vi "BITMAPINFOHEADER.vi"(11 "Dimensions de l'image":i32[](array[numeric])) -> (3 "EN-TÊTE_FICHIER_BITMAP":u8[](array[numeric]))   [LabVIEW 2009]
panel:
  out "taille(s)":i32
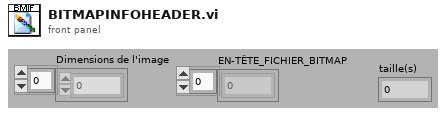
[diagram p1: front panel]
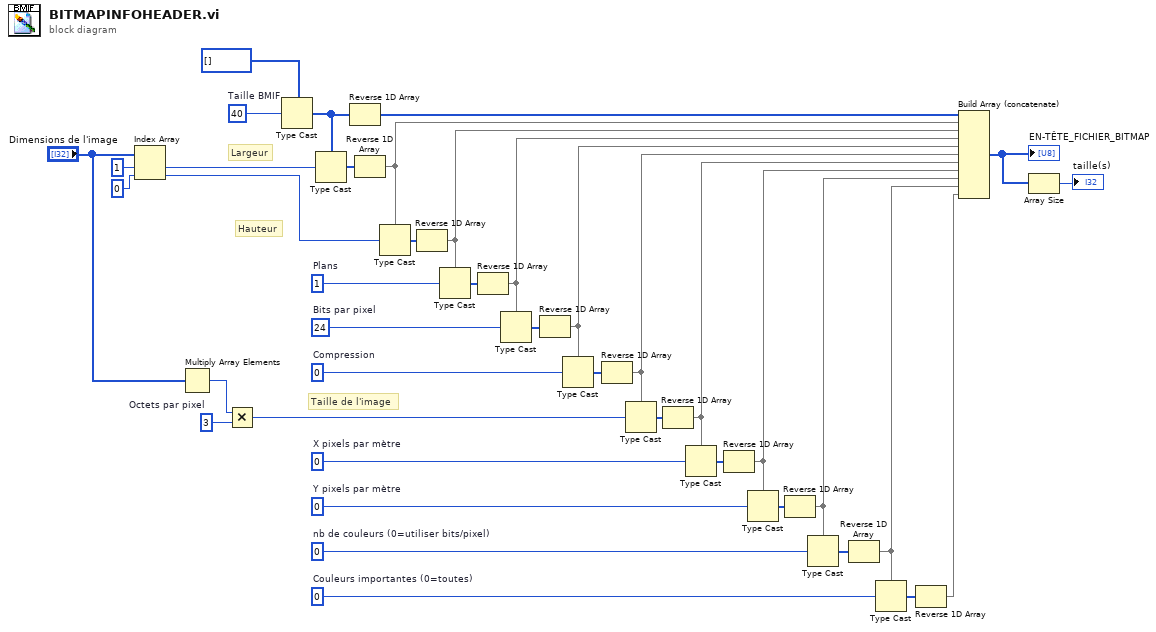
[diagram p0: block diagram]
diagram:
  w26 = 3  # Octets par pixel
  w29 = 0  # Couleurs importantes (0=toutes)
  w30 = 0  # nb de couleurs (0=utiliser bits/pixel)
  w33 = 0  # Y pixels par mètre
  w34 = 0  # X pixels par mètre
  w35 = 0  # Compression
  w36 = i16 24  # Bits par pixel
  w37 = i16 1  # Plans
  w38 = 40  # Taille BMIF
  # "Taille de l'image"
  # "Hauteur"
  # "Largeur"
  n1 = Index Array ("Indexer un tableau")(array="Dimensions de l'image", index #1=1 ("index"), index #2=0 ("index")) -> (element #1=w27:i32, element #2=w28:i32)
  n2 = Multiply Array Elements ("Multiplier les éléments du tableau")(1:"Dimensions de l'image") -> (0:w2:i32)
  n3 = Multiply ("Multiplier")(x=w2, y=w26) -> (x*y=w1:i32)
  n4 = Type Cast ("Adapter le type")(type=u8[] [], x=w38) -> (*(type *) &x=w7:u8[])
  n5 = Type Cast ("Adapter le type")(type=w7, x=w27) -> (*(type *) &x=w25:u8[])
  n6 = Reverse 1D Array ("Renverser un tableau 1D")(array=w7) -> (reversed array=w6:u8[])
  n7 = Reverse 1D Array ("Renverser un tableau 1D")(array=w25) -> (reversed array=w24:u8[])
  n8 = Type Cast ("Adapter le type")(type=w24, x=w28) -> (*(type *) &x=w23:u8[])
  n9 = Reverse 1D Array ("Renverser un tableau 1D")(array=w23) -> (reversed array=w22:u8[])
  n10 = Type Cast ("Adapter le type")(type=w22, x=w37) -> (*(type *) &x=w21:u8[])
  n11 = Reverse 1D Array ("Renverser un tableau 1D")(array=w21) -> (reversed array=w20:u8[])
  n12 = Type Cast ("Adapter le type")(type=w20, x=w36) -> (*(type *) &x=w19:u8[])
  n13 = Reverse 1D Array ("Renverser un tableau 1D")(array=w19) -> (reversed array=w18:u8[])
  n14 = Type Cast ("Adapter le type")(type=w18, x=w35) -> (*(type *) &x=w17:u8[])
  n15 = Reverse 1D Array ("Renverser un tableau 1D")(array=w17) -> (reversed array=w16:u8[])
  n16 = Type Cast ("Adapter le type")(type=w16, x=w1) -> (*(type *) &x=w15:u8[])
  n17 = Reverse 1D Array ("Renverser un tableau 1D")(array=w15) -> (reversed array=w14:u8[])
  n18 = Type Cast ("Adapter le type")(type=w14, x=w34) -> (*(type *) &x=w13:u8[])
  n19 = Reverse 1D Array ("Renverser un tableau 1D")(array=w13) -> (reversed array=w12:u8[])
  n20 = Type Cast ("Adapter le type")(type=w12, x=w33) -> (*(type *) &x=w11:u8[])
  n21 = Reverse 1D Array ("Renverser un tableau 1D")(array=w11) -> (reversed array=w10:u8[])
  n22 = Type Cast ("Adapter le type")(type=w10, x=w30) -> (*(type *) &x=w9:u8[])
  n23 = Reverse 1D Array ("Renverser un tableau 1D")(array=w9) -> (reversed array=w8:u8[])
  n24 = Type Cast ("Adapter le type")(type=w8, x=w29) -> (*(type *) &x=w5:u8[])
  n25 = Reverse 1D Array ("Renverser un tableau 1D")(array=w5) -> (reversed array=w4:u8[])
  n26 = Build Array (concatenate) ("Construire un tableau")(w6, w24, w22, w20, w18, w16, w14, w12, w10, w8, w4) -> (w32:u8[])
  "EN-TÊTE_FICHIER_BITMAP" <- w32
  n27 = Array Size ("Taille d'un tableau")(array=w32) -> (size(s)=→"taille(s)":i32)
